vi "Pixel Values Array to ARGB Data.vi"(1 "Pixel Values":u8[][][](array[numeric])) -> (0 "ARGB Data":u32[][](array[numeric]))   [LabVIEW 2020, in "g_ar_toolkit.image.lvlib"]
uses:
  g_ar_toolkit.image.lvlib
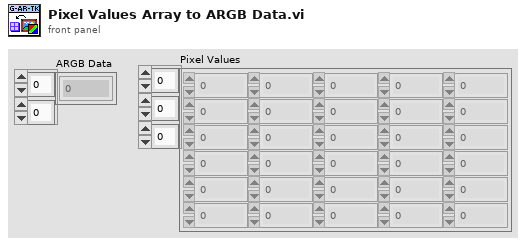
[diagram p1: front panel]
types:
  T1 = enum16{"big-endian, network order", "native, host order", "little-endian"}
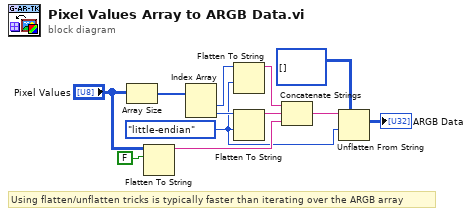
[diagram p0: block diagram]
diagram:
  w1 = T1."little-endian" ("byte order (0:big-endian, network order)")
  # "Using flatten/unflatten tricks is typically faster than iterating over the ARGB array"
  n1 = Array Size(array="Pixel Values") -> (size(s)=w5:i32[])
  n2 = Flatten To String(anything="Pixel Values", prepend array or string size? (T)=FALSE) -> (data string=w9:string)  [unwired: 2 in, 2 out]
  n3 = Index Array(array=w5) -> (element #1=w4:i32, element #2=w3:i32)  [unwired: 2 in]
  n4 = Flatten To String(anything=w4, byte order (0:big-endian, network order)=w1) -> (data string=w11:string)  [unwired: 2 in, 2 out]
  n5 = Flatten To String(anything=w3, byte order (0:big-endian, network order)=w1) -> (data string=w10:string)  [unwired: 2 in, 2 out]
  n6 = Concatenate Strings(w11, w10, w9) -> (w8:string)
  n7 = Unflatten From String(type=u32[][] [], binary string=w8, byte order (0:big-endian, network order)=w1) -> (value=→"ARGB Data":u32[][])  [unwired: 2 in, 2 out]
